vi "Classify Error.vi"(10 "Error Code":i32) -> (2 "Error Classification":u32)   [LabVIEW 2018, in "Tektronix TDS 200 1000 2000 Series.lvlib"]
doc: "This VI characterizes an error code as an error, warning, or something not of interest to the user."
uses:
  Tektronix TDS 200 1000 2000 Series.lvlib
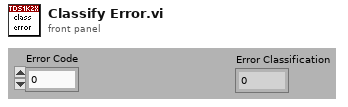
[diagram p1: front panel]
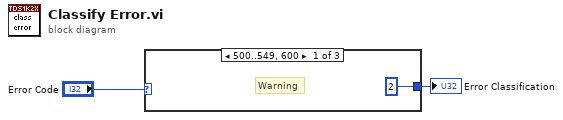
[diagram p0: block diagram]
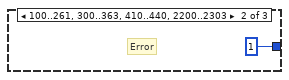
[diagram p2: hidden frame]
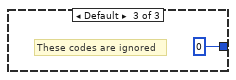
[diagram p3: hidden frame]
diagram:
  n1 = case shown="500..549, 600" "Error Code" {
    tunnel: [2 1 0] -> w1
    frame 500..549, 600 {
      # "Warning"
    }
    frame 100..261, 300..363, 410..440, 2200..2303 {
      # "Error"
    }
    frame Default {
      # "These codes are ignored"
    }
  }
  "Error Classification" <- w1
